vi "Camera Test Suite.vi"() -> ()   [LabVIEW 2018]
panel:
  out "Status":T1
  in  "Exposure":dbl=0.1
  in  "Save location":path
  out "Image":T2(plugin-control)
  in  "Test":bool
  in  "stop":bool
  in  "Function to test":T3(ring)
  in  "Camera vi path":path
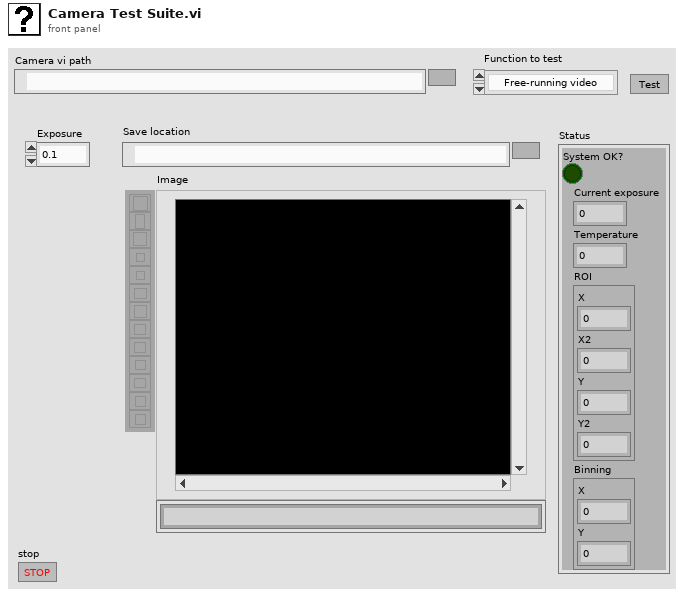
[diagram p1: front panel]
types:
  T1 = cluster{"System OK?":bool, "Current exposure":dbl, "Temperature":dbl, "ROI":cluster{"X":u32, "X2":u32, "Y":u32, "Y2":u32}, "Binning":cluster{"X":u32, "Y":u32}}
  T2 = typedef "IMAQ Image.ctl" = refnum<image>
  T3 = enum16{"Free-running video", "Capture 1 frame", "Capture 10 frames", "Settings", "Change exposure", "Get status"}
  T4 = typedef "Image Type" = u32
  T5 = enum16{"Initialize", "Shut down", "Set capture mode", "Set exposure", "Trigger and read", "Get status", "Other settings"}
  T6 = cluster{"New Image":T2, "Image":refnum<vi>, "FPS target":dbl}
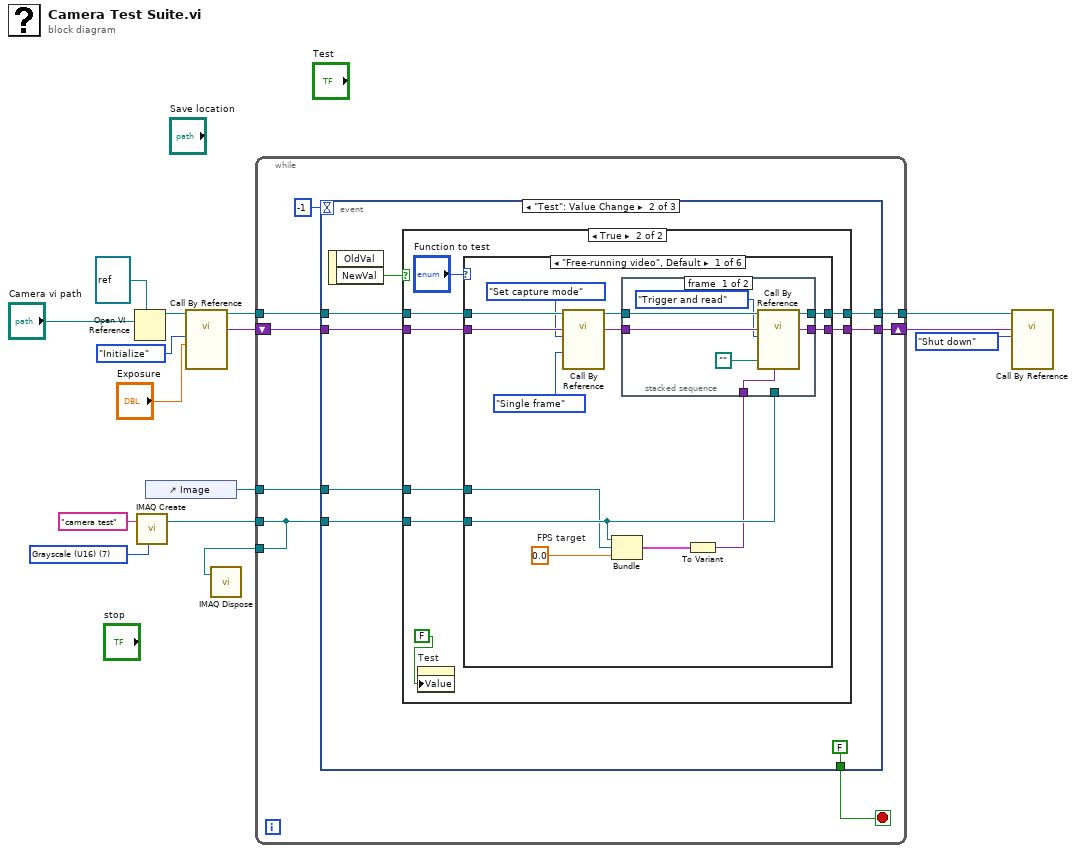
[diagram p0: block diagram]
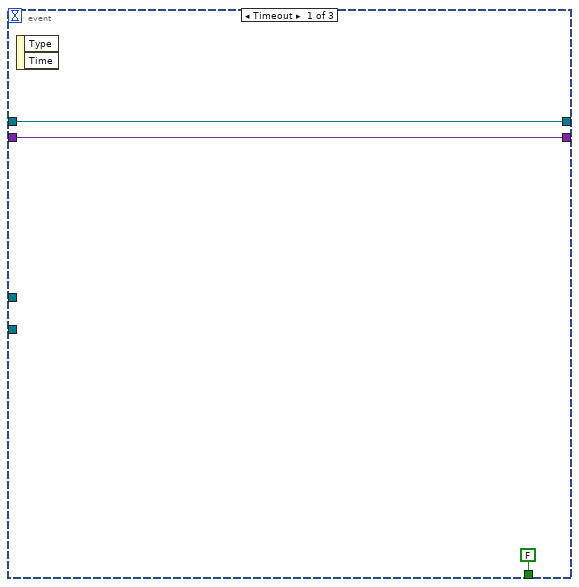
[diagram p2: hidden frame]
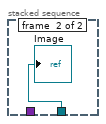
[diagram p4: hidden frame]
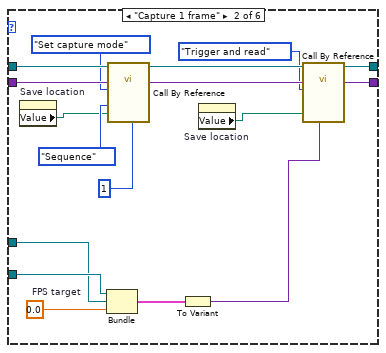
[diagram p5: hidden frame]
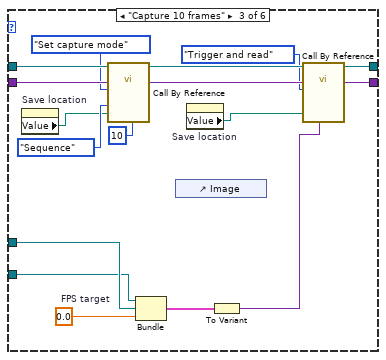
[diagram p6: hidden frame]
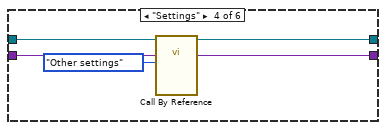
[diagram p7: hidden frame]
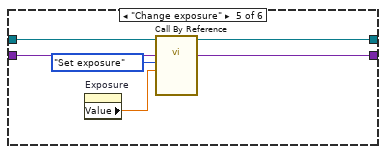
[diagram p8: hidden frame]
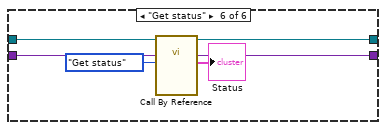
[diagram p9: hidden frame]
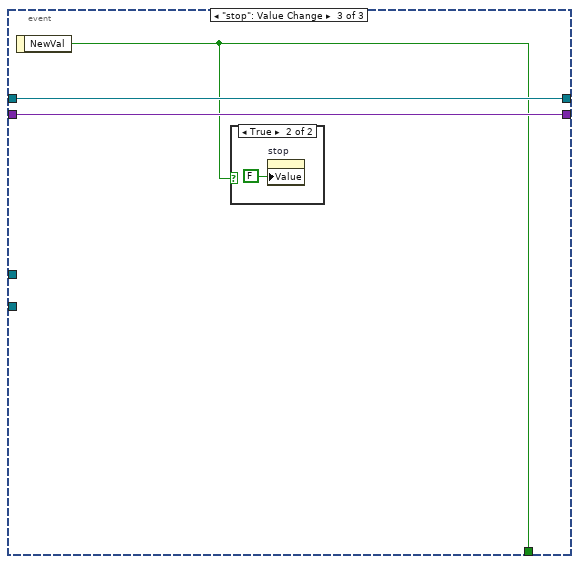
[diagram p10: hidden frame]
diagram:
  w5 = T4 7 items=["Grayscale (U8)", "Grayscale (I16)", "Grayscale (SGL)", "Complex (CSG)", "RGB (U32)", "HSL (U32)", "RGB (U64)", "Grayscale (U16)"] ("Image Type")
  n1 = Open VI Reference(type specifier VI Refnum (for type only)=refnum<vi> refnum, vi path="Camera vi path") -> (vi reference=w13:refnum<vi>)  [unwired: 4 in, 1 out]
  n2 = call "IMAQ Create"("Image Name"="camera test", "Image Type"=w5) -> ("New Image"=w4:T2)  [unwired: 3 in, 1 out]
  n3 = control-ref of="Image"() -> (w1:refnum<vi>)
  n4 = call-by-ref "?"(reference=w13, "Exposure time (s)"="Exposure", "Operation"=T5."Initialize") -> (reference out=w10:refnum<vi>, "Camera-specific out"=w8:variant)  [unwired: 9 in, 2 out]
  n5 = while {
    tunnel: w10 -> [w21]
    tunnel: [w22] -> w12
    shift-right: [w20] -> w7
    shift-left: w8 -> [w19]
    tunnel: w4 -> [w18]
    tunnel: [w18] -> w3
    tunnel: w1 -> [w16]
    stop <- w17 stop-if-true
    n6 = event shown="[1] \"Test\": Value Change" {
      selector: _ -> [_ _ _]
      dyn-events: _ -> [_ _ _]
      timeout: -1 -> [_ _ _]
      tunnel: [w26 w34 w119] -> w22
      tunnel: w21 -> [w26 w33 w119]
      tunnel: [w25 w32 w118] -> w20
      tunnel: w19 -> [w25 w31 w118]
      tunnel: w18 -> [_ w29 _]
      tunnel: [FALSE ("NewVal") FALSE ("NewVal") w117] -> w17
      tunnel: w16 -> [_ w27 _]
      event Timeout {
        n7 = event-data() -> ()  [unwired: 1 in, 2 out]
      }
      event "Test": Value Change {
        n8 = event-data() -> ("NewVal"=w30:bool)  [unwired: 1 in, 1 out]
        n9 = case shown="True" w30 {
          tunnel: [w36 w43] -> w34
          tunnel: w33 -> [w36 w42]
          tunnel: [w35 w41] -> w32
          tunnel: w31 -> [w35 w40]
          tunnel: w29 -> [_ w38]
          tunnel: w27 -> [_ w37]
          frame False {
          }
          frame True {
            n10 = property on="Test" class="Bool (strict)"("Value"=FALSE) -> ()  [unwired: 2 in, 2 out]
            n11 = case shown="\"Free-running video\", Default" "Function to test" {
              tunnel: [w52 w77 w94 w103 w109 w115] -> w43
              tunnel: w42 -> [w57 w82 w99 w104 w110 w116]
              tunnel: [w50 w75 w92 w101 w107 w113] -> w41
              tunnel: w40 -> [w56 w81 w98 w102 w108 w114]
              tunnel: w38 -> [w47 w72 w86 _ _ _]
              tunnel: w37 -> [w46 w71 w87 _ _ _]
              frame "Free-running video", Default {
                w49 = 0.0  # FPS target
                n12 = call-by-ref "?"(reference=w57, "Camera-specific in"=w56, "Capture mode"=enum16{"Single frame", "Sequence"}."Single frame", "Operation"=T5."Set capture mode") -> (reference out=w53:refnum<vi>, "Camera-specific out"=w51:variant)  [unwired: 8 in, 2 out]
                n13 = Bundle("New Image"=w47, "Image"=w46, "FPS target"=w49) -> (w48:T6)  [unwired: 1 in]
                n14 = To Variant(anything=w48) -> (Variant=w45:variant)
                n15 = stacked-sequence {
                  tunnel: w53 -> [w64 _]
                  tunnel: [w63 _] -> w52
                  tunnel: w51 -> [w62 _]
                  tunnel: [w61 _] -> w50
                  tunnel: w47 -> [_ w65]
                  tunnel: w45 -> [w58 _]
                  frame #0 {
                    n16 = call-by-ref "?"(reference=w64, "Image in"=w58, "Camera-specific in"=w62, "Save path"=path "", "Operation"=T5."Trigger and read") -> (reference out=w63:refnum<vi>, "Camera-specific out"=w61:variant)  [unwired: 7 in, 2 out]
                  }
                  frame #1 {
                    "Image" <- w65
                  }
                }
              }
              frame "Capture 1 frame" {
                w70 = 0.0  # FPS target
                n17 = property on="Save location" class="Path"() -> ("Value"=w73:path)  [unwired: 2 in, 2 out]
                n18 = Bundle("New Image"=w72, "Image"=w71, "FPS target"=w70) -> (w69:T6)  [unwired: 1 in]
                n19 = call-by-ref "?"(reference=w82, "Frames in sequence"=u32 1, "Camera-specific in"=w81, "Save path"=w73, "Capture mode"=enum16{"Single frame", "Sequence"}."Sequence", "Operation"=T5."Set capture mode") -> (reference out=w78:refnum<vi>, "Camera-specific out"=w76:variant)  [unwired: 6 in, 2 out]
                n20 = To Variant(anything=w69) -> (Variant=w68:variant)
                n21 = property on="Save location" class="Path"() -> ("Value"=w66:path)  [unwired: 2 in, 2 out]
                n22 = call-by-ref "?"(reference=w78, "Image in"=w68, "Camera-specific in"=w76, "Save path"=w66, "Operation"=T5."Trigger and read") -> (reference out=w77:refnum<vi>, "Camera-specific out"=w75:variant)  [unwired: 7 in, 2 out]
              }
              frame "Capture 10 frames" {
                w89 = 0.0  # FPS target
                n23 = property on="Save location" class="Path"() -> ("Value"=w90:path)  [unwired: 2 in, 2 out]
                n24 = call-by-ref "?"(reference=w99, "Frames in sequence"=u32 10, "Camera-specific in"=w98, "Save path"=w90, "Capture mode"=enum16{"Single frame", "Sequence"}."Sequence", "Operation"=T5."Set capture mode") -> (reference out=w95:refnum<vi>, "Camera-specific out"=w93:variant)  [unwired: 6 in, 2 out]
                n25 = Bundle("New Image"=w86, "Image"=w87, "FPS target"=w89) -> (w88:T6)  [unwired: 1 in]
                n26 = control-ref of="Image"() -> ()  [unwired: 1 out]
                n27 = property on="Save location" class="Path"() -> ("Value"=w83:path)  [unwired: 2 in, 2 out]
                n28 = To Variant(anything=w88) -> (Variant=w85:variant)
                n29 = call-by-ref "?"(reference=w95, "Image in"=w85, "Camera-specific in"=w93, "Save path"=w83, "Operation"=T5."Trigger and read") -> (reference out=w94:refnum<vi>, "Camera-specific out"=w92:variant)  [unwired: 7 in, 2 out]
              }
              frame "Settings" {
                n30 = call-by-ref "?"(reference=w104, "Camera-specific in"=w102, "Operation"=T5."Other settings") -> (reference out=w103:refnum<vi>, "Camera-specific out"=w101:variant)  [unwired: 9 in, 2 out]
              }
              frame "Change exposure" {
                n31 = property on="Exposure" class="DigNum (strict)"() -> ("Value"=w105:dbl)  [unwired: 2 in, 2 out]
                n32 = call-by-ref "?"(reference=w110, "Camera-specific in"=w108, "Exposure time (s)"=w105, "Operation"=T5."Set exposure") -> (reference out=w109:refnum<vi>, "Camera-specific out"=w107:variant)  [unwired: 8 in, 2 out]
              }
              frame "Get status" {
                n33 = call-by-ref "?"(reference=w116, "Camera-specific in"=w114, "Operation"=T5."Get status") -> (reference out=w115:refnum<vi>, "Status"=→"Status":T1, "Camera-specific out"=w113:variant)  [unwired: 9 in, 1 out]
              }
            }
          }
        }
      }
      event "stop": Value Change {
        n34 = event-data() -> ("NewVal"=w117:bool)  [unwired: 1 in]
        n35 = case shown="True" w117 {
          frame False {
          }
          frame True {
            n36 = property on="stop" class="Bool (strict)"("Value"=FALSE ("stop")) -> ()  [unwired: 2 in, 2 out]
          }
        }
      }
    }
  }
  n37 = call "IMAQ Dispose"("Image"=w3) -> ()  [unwired: 5 in, 1 out]
  n38 = call-by-ref "?"(reference=w12, "Camera-specific in"=w7, "Operation"=T5."Shut down") -> ()  [unwired: 9 in, 4 out]
